vi "_WriteSubData_TDMS_ALTIMETER.vi"(8 "error in (no error)":errorcluster, 10 "Sub Data in":T1 {"Control"."motor_ctrl_array"."sensor" format="%#.2f"; "Control"."motor_ctrl_array"."setpoint" format="%#.2f"; "Control"."dac_outputs" format="%#.2f"; "PWR"."motor_array"."motor_name" items=["Motor1", "Motor2", "Motor3", "Motor4", "Motor5", "Motor6"]}, 11 "Refnum in":refnum<k34>) -> (0 "error out":errorcluster, 3 "Refnum out":refnum<k34>)   [LabVIEW 2018]
uses:
  TypeDefsSubsea/Sub Data.ctl
  TypeDefsSubsea/Sub Status.ctl
  Shared/Type Defs/ROV States.ctl
  Shared/Type Defs/SMP.ctl
  Shared/Type Defs/PWR.ctl
  Shared/Type Defs/Motor.ctl
  Shared/Type Defs/MotorNames.ctl
  Shared/Type Defs/SmartCard.ctl
  Shared/Type Defs/Box Names.ctl
  TypeDefsSubsea/Sub Control.ctl
  TypeDefsSubsea/Modos Control.ctl
  TypeDefsSubsea/ROV Outputs.ctl
  TypeDefsSubsea/Motor Control.ctl
  TypeDefsSubsea/Type Defs Subsea.lvlib
  TypeDefsTopside/Type Defs Topside.lvlib
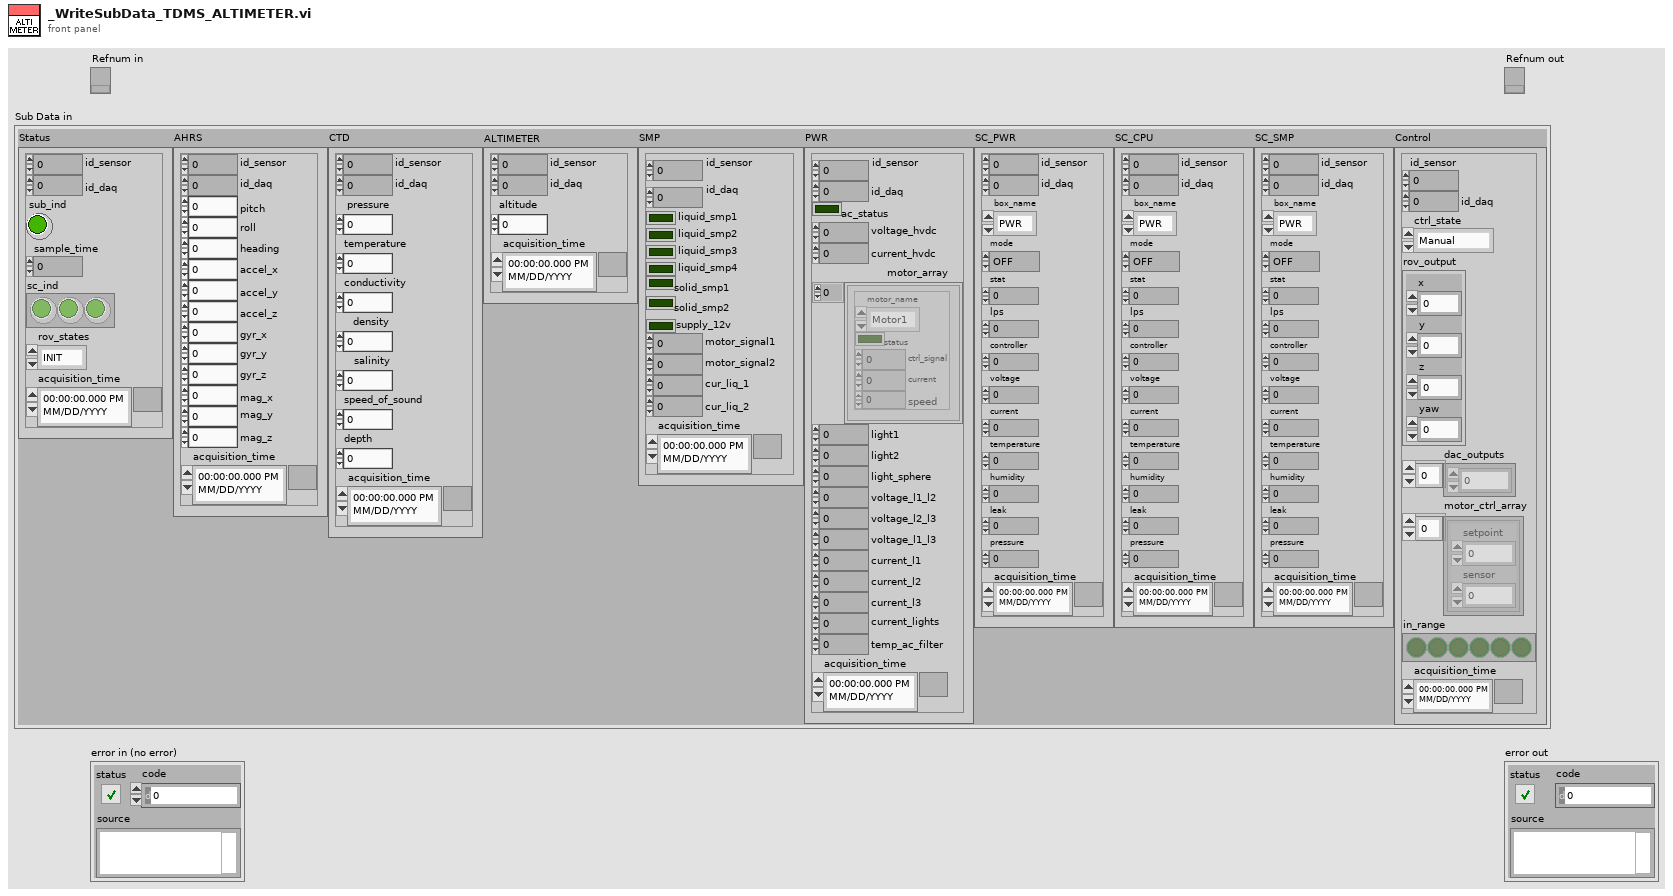
[diagram p1: front panel]
types:
  T1 = typedef "Type Defs Subsea.lvlib/Sub Data.ctl" = cluster{"Status":T2, "AHRS":cluster{"id_sensor":u32, "id_daq":u64, "pitch":dbl, "roll":dbl, "heading":dbl, "accel_x":dbl, "accel_y":dbl, "accel_z":dbl, "gyr_x":dbl, "gyr_y":dbl, "gyr_z":dbl, "mag_x":dbl, "mag_y":dbl, "mag_z":dbl, "acquisition_time":timestamp}, "CTD":cluster{"id_sensor":u32, "id_daq":u64, "pressure":dbl, "temperature":dbl, "conductivity":dbl, "density":dbl, "salinity":dbl, "speed_of_sound":dbl, "depth":dbl, "acquisition_time":timestamp}, "ALTIMETER":cluster{"id_sensor":u32, "id_daq":u64, "altitude":dbl, "acquisition_time":timestamp}, "SMP":T4, "PWR":T5, "SC_PWR":T8, "SC_CPU":T8, "SC_SMP":T8, "Control":T10}
  T2 = typedef "Type Defs Subsea.lvlib/Sub Status.ctl" = cluster{"id_sensor":u32, "id_daq":u32, "sub_ind":bool, "sample_time":i64, "sc_ind":bool[], "rov_states":T3, "acquisition_time":timestamp}
  T3 = typedef "Type Defs Subsea.lvlib/ROV States.ctl" = enum16{"INIT", "IDLE", "TEST", "RUN", "EMERGENCY", "EXIT"}
  T4 = typedef "Type Defs Subsea.lvlib/SMP.ctl" = cluster{"id_sensor":u32, "id_daq":u64, "liquid_smp1":bool, "liquid_smp2":bool, "liquid_smp3":bool, "liquid_smp4":bool, "solid_smp1":bool, "solid_smp2":bool, "supply_12v":bool, "motor_signal1":dbl, "motor_signal2":dbl, "cur_liq_1":dbl, "cur_liq_2":dbl, "acquisition_time":timestamp}
  T5 = typedef "Type Defs Topside.lvlib/PWR.ctl" = cluster{"id_sensor":u32, "id_daq":u64, "ac_status":bool, "voltage_hvdc":dbl, "current_hvdc":dbl, "motor_array":T6[], "light1":dbl, "light2":dbl, "light_sphere":dbl, "voltage_l1_l2":dbl, "voltage_l2_l3":dbl, "voltage_l1_l3":dbl, "current_l1":dbl, "current_l2":dbl, "current_l3":dbl, "current_lights":dbl, "temp_ac_filter":dbl, "acquisition_time":timestamp}
  T6 = typedef "Type Defs Subsea.lvlib/Motor.ctl" = cluster{"motor_name":T7, "status":bool, "ctrl_signal":dbl, "current":dbl, "speed":dbl}
  T7 = typedef "Type Defs Subsea.lvlib/MotorNames.ctl" = u16
  T8 = typedef "Type Defs Subsea.lvlib/SmartCard.ctl" = cluster{"id_sensor":u32, "id_daq":u64, "box_name":T9, "mode":enum16{"OFF", "STANDBY", "TESTING", "RUN", "EMERGENCY"}, "stat":dbl, "lps":dbl, "controller":dbl, "voltage":dbl, "current":dbl, "temperature":dbl, "humidity":dbl, "leak":dbl, "pressure":dbl, "acquisition_time":timestamp}
  T9 = typedef "Type Defs Subsea.lvlib/Box Names.ctl" = enum16{"PWR", "CPU", "SMP"}
  T10 = typedef "Type Defs Subsea.lvlib/Sub Control.ctl" = cluster{"id_sensor":u32, "id_daq":u64, "ctrl_state":T11, "rov_output":T12, "dac_outputs":dbl[], "motor_ctrl_array":T13[], "in_range":bool[], "acquisition_time":timestamp}
  T11 = typedef "Type Defs Subsea.lvlib/Modos Control.ctl" = enum16{"Manual", "Profundidad", "Altitud", "Rumbo", "P+R"}
  T12 = typedef "Type Defs Subsea.lvlib/ROV Outputs.ctl" = cluster{"x":dbl, "y":dbl, "z":dbl, "yaw":dbl}
  T13 = typedef "Type Defs Subsea.lvlib/Motor Control.ctl" = cluster{"setpoint":dbl, "sensor":dbl}
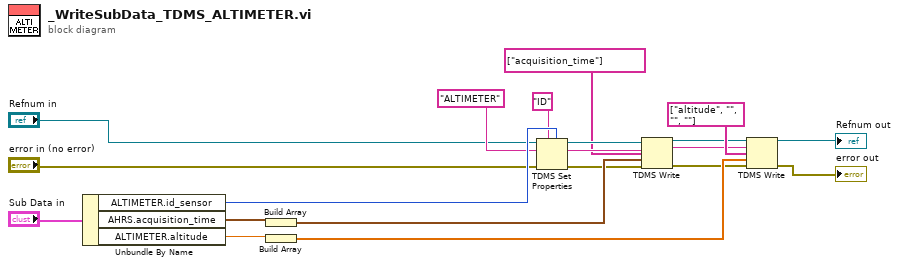
[diagram p0: block diagram]
diagram:
  n1 = Unbundle By Name("Sub Data in") -> ("ALTIMETER.id_sensor"=w16:u32, "AHRS.acquisition_time"=w17:timestamp, "ALTIMETER.altitude"=w18:dbl)
  n2 = Build Array(w17) -> (w19:timestamp[])
  n3 = Build Array(w18) -> (w20:dbl[])
  n4 = TDMS Set Properties(5:w16, 7:"ID" ("property names"), 8:"error in (no error)", 10:"ALTIMETER" ("group name in (Untitled)"), 11:"Refnum in") -> (0:w15:errorcluster, 2:w14:string, 3:w12:refnum<k34>)  [unwired: 1 in, 1 out]
  n5 = TDMS Write(0:w12, 5:w14, 7:string[] ["acquisition_time"] ("channel name(s) in (Untitled)"), 9:w19, 11:w15) -> (4:w8:refnum<k34>, 6:w7:string, 15:w9:errorcluster)  [unwired: 1 in, 1 out]
  n6 = TDMS Write(0:w8, 5:w7, 7:string[] ["altitude", "", "", ""] ("channel name(s) in (Untitled)"), 9:w20, 11:w9) -> (4:→"Refnum out":refnum<k34>, 15:→"error out":errorcluster)  [unwired: 1 in, 2 out]
